vi "subvi_corrdinate.vi"(7 "current puzzle":picture[][](array[picture]), 9 "2D Picture":picture) -> (2 "white location":cluster{i32, i32}, 3 "piece location":cluster{i32, i32})   [LabVIEW 2014]
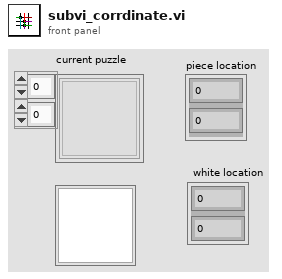
[diagram p1: front panel]
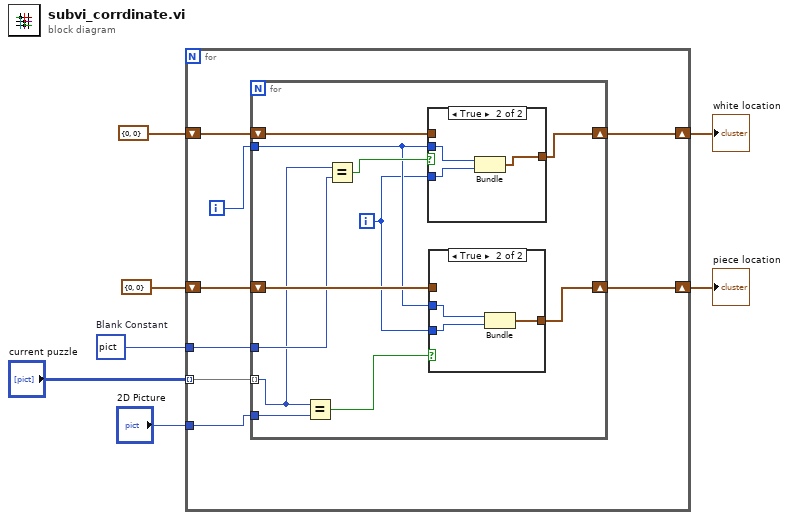
[diagram p0: block diagram]
diagram:
  w6 = picture data[5B]  # Blank Constant
  n1 = for {
    shift-right: [w9] -> w2
    shift-left: cluster{i32, i32} {0, 0} -> [w15]
    tunnel: w6 -> [w12]
    shift-right: [w8] -> w1
    shift-left: cluster{i32, i32} {0, 0} -> [w14]
    tunnel: "current puzzle" -> [w13] mode=indexing
    tunnel: "2D Picture" -> [w11]
    i -> [w10]
    n2 = for {
      shift-right: [w17] -> w9
      shift-left: w15 -> [w26]
      shift-right: [w16] -> w8
      shift-left: w14 -> [w25]
      tunnel: w13 -> [w21] mode=indexing
      tunnel: w12 -> [w22]
      tunnel: w11 -> [w23]
      tunnel: w10 -> [w19]
      i -> [w18]
      n3 = Equal?(x=w21, y=w23) -> (x = y?=w24:bool)
      n4 = Equal?(x=w21, y=w22) -> (x = y?=w20:bool)
      n5 = case shown="True" w20 {
        tunnel: w26 -> [w31 _]
        tunnel: w19 -> [_ w34]
        tunnel: w18 -> [_ w33]
        tunnel: [w31 w32] -> w17
        frame False {
        }
        frame True {
          n6 = Bundle(w34, w33) -> (w32:cluster{i32, i32})  [unwired: 1 in]
        }
      }
      n7 = case shown="True" w24 {
        tunnel: w25 -> [w27 _]
        tunnel: w19 -> [_ w30]
        tunnel: w18 -> [_ w29]
        tunnel: [w27 w28] -> w16
        frame False {
        }
        frame True {
          n8 = Bundle(w30, w29) -> (w28:cluster{i32, i32})  [unwired: 1 in]
        }
      }
    }
  }
  "white location" <- w2
  "piece location" <- w1
